vi "polymorphic_addation.vi"   [LabVIEW 2020]
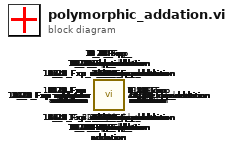
[diagram p0: block diagram]
diagram:
  n1 = call "16_32_Fxp_addation.vi"() -> ()  [unwired: 2 in, 1 out]
  n2 = call "15_32_Fxp_addation.vi"() -> ()  [unwired: 2 in, 1 out]
  n3 = call "14_32_Fxp_addation.vi"() -> ()  [unwired: 2 in, 1 out]
  n4 = call "13_32_Fxp_addation.vi"() -> ()  [unwired: 2 in, 1 out]
  n5 = call "12_32_Fxp_addation.vi"() -> ()  [unwired: 2 in, 1 out]
  n6 = call "11_32_Fxp_addation.vi"() -> ()  [unwired: 2 in, 1 out]
  n7 = call "10_32_Fxp_addation.vi"() -> ()  [unwired: 2 in, 1 out]
  n8 = call "9_32_Fxp_addation.vi"() -> ()  [unwired: 2 in, 1 out]
  n9 = call "8_32_Fxp_addation.vi"() -> ()  [unwired: 2 in, 1 out]
  n10 = call "7_32_Fxp_addation.vi"() -> ()  [unwired: 2 in, 1 out]
  n11 = call "6_32_Fxp_addation.vi"() -> ()  [unwired: 2 in, 1 out]
  n12 = call "5_32_Fxp_addation.vi"() -> ()  [unwired: 2 in, 1 out]
  n13 = call "4_32_Fxp_addation.vi"() -> ()  [unwired: 2 in, 1 out]
  n14 = call "3_32_Fxp_addation.vi"() -> ()  [unwired: 2 in, 1 out]
  n15 = call "2_32_Fxp_addation.vi"() -> ()  [unwired: 2 in, 1 out]
  n16 = call "1_32_Fxp_addation.vi"() -> ()  [unwired: 2 in, 1 out]
  n17 = call "16_31_Fxp_addation.vi"() -> ()  [unwired: 2 in, 1 out]
  n18 = call "15_31_Fxp_addation.vi"() -> ()  [unwired: 2 in, 1 out]
  n19 = call "14_31_Fxp_addation.vi"() -> ()  [unwired: 2 in, 1 out]
  n20 = call "13_31_Fxp_addation.vi"() -> ()  [unwired: 2 in, 1 out]
  n21 = call "12_31_Fxp_addation.vi"() -> ()  [unwired: 2 in, 1 out]
  n22 = call "11_31_Fxp_addation.vi"() -> ()  [unwired: 2 in, 1 out]
  n23 = call "10_31_Fxp_addation.vi"() -> ()  [unwired: 2 in, 1 out]
  n24 = call "9_31_Fxp_addation.vi"() -> ()  [unwired: 2 in, 1 out]
  n25 = call "8_31_Fxp_addation.vi"() -> ()  [unwired: 2 in, 1 out]
  n26 = call "7_31_Fxp_addation.vi"() -> ()  [unwired: 2 in, 1 out]
  n27 = call "6_31_Fxp_addation.vi"() -> ()  [unwired: 2 in, 1 out]
  n28 = call "5_31_Fxp_addation.vi"() -> ()  [unwired: 2 in, 1 out]
  n29 = call "4_31_Fxp_addation.vi"() -> ()  [unwired: 2 in, 1 out]
  n30 = call "3_31_Fxp_addation.vi"() -> ()  [unwired: 2 in, 1 out]
  n31 = call "2_31_Fxp_addation.vi"() -> ()  [unwired: 2 in, 1 out]
  n32 = call "1_31_Fxp_addation.vi"() -> ()  [unwired: 2 in, 1 out]
  n33 = call "16_30_Fxp_addation.vi"() -> ()  [unwired: 2 in, 1 out]
  n34 = call "15_30_Fxp_addation.vi"() -> ()  [unwired: 2 in, 1 out]
  n35 = call "14_30_Fxp_addation.vi"() -> ()  [unwired: 2 in, 1 out]
  n36 = call "13_30_Fxp_addation.vi"() -> ()  [unwired: 2 in, 1 out]
  n37 = call "12_30_Fxp_addation.vi"() -> ()  [unwired: 2 in, 1 out]
  n38 = call "11_30_Fxp_addation.vi"() -> ()  [unwired: 2 in, 1 out]
  n39 = call "10_30_Fxp_addation.vi"() -> ()  [unwired: 2 in, 1 out]
  n40 = call "9_30_Fxp_addation.vi"() -> ()  [unwired: 2 in, 1 out]
  n41 = call "8_30_Fxp_addation.vi"() -> ()  [unwired: 2 in, 1 out]
  n42 = call "7_30_Fxp_addation.vi"() -> ()  [unwired: 2 in, 1 out]
  n43 = call "6_30_Fxp_addation.vi"() -> ()  [unwired: 2 in, 1 out]
  n44 = call "5_30_Fxp_addation.vi"() -> ()  [unwired: 2 in, 1 out]
  n45 = call "4_30_Fxp_addation.vi"() -> ()  [unwired: 2 in, 1 out]
  n46 = call "3_30_Fxp_addation.vi"() -> ()  [unwired: 2 in, 1 out]
  n47 = call "2_30_Fxp_addation.vi"() -> ()  [unwired: 2 in, 1 out]
  n48 = call "1_30_Fxp_addation.vi"() -> ()  [unwired: 2 in, 1 out]
  n49 = call "16_29_Fxp_addation.vi"() -> ()  [unwired: 2 in, 1 out]
  n50 = call "15_29_Fxp_addation.vi"() -> ()  [unwired: 2 in, 1 out]
  n51 = call "14_29_Fxp_addation.vi"() -> ()  [unwired: 2 in, 1 out]
  n52 = call "13_29_Fxp_addation.vi"() -> ()  [unwired: 2 in, 1 out]
  n53 = call "12_29_Fxp_addation.vi"() -> ()  [unwired: 2 in, 1 out]
  n54 = call "11_29_Fxp_addation.vi"() -> ()  [unwired: 2 in, 1 out]
  n55 = call "10_29_Fxp_addation.vi"() -> ()  [unwired: 2 in, 1 out]
  n56 = call "9_29_Fxp_addation.vi"() -> ()  [unwired: 2 in, 1 out]
  n57 = call "8_29_Fxp_addation.vi"() -> ()  [unwired: 2 in, 1 out]
  n58 = call "7_29_Fxp_addation.vi"() -> ()  [unwired: 2 in, 1 out]
  n59 = call "6_29_Fxp_addation.vi"() -> ()  [unwired: 2 in, 1 out]
  n60 = call "5_29_Fxp_addation.vi"() -> ()  [unwired: 2 in, 1 out]
  n61 = call "4_29_Fxp_addation.vi"() -> ()  [unwired: 2 in, 1 out]
  n62 = call "3_29_Fxp_addation.vi"() -> ()  [unwired: 2 in, 1 out]
  n63 = call "2_29_Fxp_addation.vi"() -> ()  [unwired: 2 in, 1 out]
  n64 = call "1_29_Fxp_addation.vi"() -> ()  [unwired: 2 in, 1 out]
  n65 = call "16_28_Fxp_addation.vi"() -> ()  [unwired: 2 in, 1 out]
  n66 = call "15_28_Fxp_addation.vi"() -> ()  [unwired: 2 in, 1 out]
  n67 = call "14_28_Fxp_addation.vi"() -> ()  [unwired: 2 in, 1 out]
  n68 = call "13_28_Fxp_addation.vi"() -> ()  [unwired: 2 in, 1 out]
  n69 = call "12_28_Fxp_addation.vi"() -> ()  [unwired: 2 in, 1 out]
  n70 = call "11_28_Fxp_addation.vi"() -> ()  [unwired: 2 in, 1 out]
  n71 = call "10_28_Fxp_addation.vi"() -> ()  [unwired: 2 in, 1 out]
  n72 = call "9_28_Fxp_addation.vi"() -> ()  [unwired: 2 in, 1 out]
  n73 = call "8_28_Fxp_addation.vi"() -> ()  [unwired: 2 in, 1 out]
  n74 = call "7_28_Fxp_addation.vi"() -> ()  [unwired: 2 in, 1 out]
  n75 = call "6_28_Fxp_addation.vi"() -> ()  [unwired: 2 in, 1 out]
  n76 = call "5_28_Fxp_addation.vi"() -> ()  [unwired: 2 in, 1 out]
  n77 = call "4_28_Fxp_addation.vi"() -> ()  [unwired: 2 in, 1 out]
  n78 = call "3_28_Fxp_addation.vi"() -> ()  [unwired: 2 in, 1 out]
  n79 = call "2_28_Fxp_addation.vi"() -> ()  [unwired: 2 in, 1 out]
  n80 = call "1_28_Fxp_addation.vi"() -> ()  [unwired: 2 in, 1 out]
  n81 = call "16_27_Fxp_addation.vi"() -> ()  [unwired: 2 in, 1 out]
  n82 = call "15_27_Fxp_addation.vi"() -> ()  [unwired: 2 in, 1 out]
  n83 = call "14_27_Fxp_addation.vi"() -> ()  [unwired: 2 in, 1 out]
  n84 = call "13_27_Fxp_addation.vi"() -> ()  [unwired: 2 in, 1 out]
  n85 = call "12_27_Fxp_addation.vi"() -> ()  [unwired: 2 in, 1 out]
  n86 = call "11_27_Fxp_addation.vi"() -> ()  [unwired: 2 in, 1 out]
  n87 = call "10_27_Fxp_addation.vi"() -> ()  [unwired: 2 in, 1 out]
  n88 = call "9_27_Fxp_addation.vi"() -> ()  [unwired: 2 in, 1 out]
  n89 = call "8_27_Fxp_addation.vi"() -> ()  [unwired: 2 in, 1 out]
  n90 = call "7_27_Fxp_addation.vi"() -> ()  [unwired: 2 in, 1 out]
  n91 = call "6_27_Fxp_addation.vi"() -> ()  [unwired: 2 in, 1 out]
  n92 = call "5_27_Fxp_addation.vi"() -> ()  [unwired: 2 in, 1 out]
  n93 = call "4_27_Fxp_addation.vi"() -> ()  [unwired: 2 in, 1 out]
  n94 = call "3_27_Fxp_addation.vi"() -> ()  [unwired: 2 in, 1 out]
  n95 = call "2_27_Fxp_addation.vi"() -> ()  [unwired: 2 in, 1 out]
  n96 = call "1_27_Fxp_addation.vi"() -> ()  [unwired: 2 in, 1 out]
  n97 = call "16_26_Fxp_addation.vi"() -> ()  [unwired: 2 in, 1 out]
  n98 = call "15_26_Fxp_addation.vi"() -> ()  [unwired: 2 in, 1 out]
  n99 = call "14_26_Fxp_addation.vi"() -> ()  [unwired: 2 in, 1 out]
  n100 = call "13_26_Fxp_addation.vi"() -> ()  [unwired: 2 in, 1 out]
  n101 = call "12_26_Fxp_addation.vi"() -> ()  [unwired: 2 in, 1 out]
  n102 = call "11_26_Fxp_addation.vi"() -> ()  [unwired: 2 in, 1 out]
  n103 = call "10_26_Fxp_addation.vi"() -> ()  [unwired: 2 in, 1 out]
  n104 = call "9_26_Fxp_addation.vi"() -> ()  [unwired: 2 in, 1 out]
  n105 = call "8_26_Fxp_addation.vi"() -> ()  [unwired: 2 in, 1 out]
  n106 = call "7_26_Fxp_addation.vi"() -> ()  [unwired: 2 in, 1 out]
  n107 = call "6_26_Fxp_addation.vi"() -> ()  [unwired: 2 in, 1 out]
  n108 = call "5_26_Fxp_addation.vi"() -> ()  [unwired: 2 in, 1 out]
  n109 = call "4_26_Fxp_addation.vi"() -> ()  [unwired: 2 in, 1 out]
  n110 = call "3_26_Fxp_addation.vi"() -> ()  [unwired: 2 in, 1 out]
  n111 = call "2_26_Fxp_addation.vi"() -> ()  [unwired: 2 in, 1 out]
  n112 = call "1_26_Fxp_addation.vi"() -> ()  [unwired: 2 in, 1 out]
  n113 = call "16_25_Fxp_addation.vi"() -> ()  [unwired: 2 in, 1 out]
  n114 = call "15_25_Fxp_addation.vi"() -> ()  [unwired: 2 in, 1 out]
  n115 = call "14_25_Fxp_addation.vi"() -> ()  [unwired: 2 in, 1 out]
  n116 = call "13_25_Fxp_addation.vi"() -> ()  [unwired: 2 in, 1 out]
  n117 = call "12_25_Fxp_addation.vi"() -> ()  [unwired: 2 in, 1 out]
  n118 = call "11_25_Fxp_addation.vi"() -> ()  [unwired: 2 in, 1 out]
  n119 = call "10_25_Fxp_addation.vi"() -> ()  [unwired: 2 in, 1 out]
  n120 = call "9_25_Fxp_addation.vi"() -> ()  [unwired: 2 in, 1 out]
  n121 = call "8_25_Fxp_addation.vi"() -> ()  [unwired: 2 in, 1 out]
  n122 = call "7_25_Fxp_addation.vi"() -> ()  [unwired: 2 in, 1 out]
  n123 = call "6_25_Fxp_addation.vi"() -> ()  [unwired: 2 in, 1 out]
  n124 = call "5_25_Fxp_addation.vi"() -> ()  [unwired: 2 in, 1 out]
  n125 = call "4_25_Fxp_addation.vi"() -> ()  [unwired: 2 in, 1 out]
  n126 = call "3_25_Fxp_addation.vi"() -> ()  [unwired: 2 in, 1 out]
  n127 = call "2_25_Fxp_addation.vi"() -> ()  [unwired: 2 in, 1 out]
  n128 = call "1_25_Fxp_addation.vi"() -> ()  [unwired: 2 in, 1 out]
  n129 = call "16_24_Fxp_addation.vi"() -> ()  [unwired: 2 in, 1 out]
  n130 = call "15_24_Fxp_addation.vi"() -> ()  [unwired: 2 in, 1 out]
  n131 = call "14_24_Fxp_addation.vi"() -> ()  [unwired: 2 in, 1 out]
  n132 = call "13_24_Fxp_addation.vi"() -> ()  [unwired: 2 in, 1 out]
  n133 = call "12_24_Fxp_addation.vi"() -> ()  [unwired: 2 in, 1 out]
  n134 = call "11_24_Fxp_addation.vi"() -> ()  [unwired: 2 in, 1 out]
  n135 = call "10_24_Fxp_addation.vi"() -> ()  [unwired: 2 in, 1 out]
  n136 = call "9_24_Fxp_addation.vi"() -> ()  [unwired: 2 in, 1 out]
  n137 = call "8_24_Fxp_addation.vi"() -> ()  [unwired: 2 in, 1 out]
  n138 = call "7_24_Fxp_addation.vi"() -> ()  [unwired: 2 in, 1 out]
  n139 = call "6_24_Fxp_addation.vi"() -> ()  [unwired: 2 in, 1 out]
  n140 = call "5_24_Fxp_addation.vi"() -> ()  [unwired: 2 in, 1 out]
  n141 = call "4_24_Fxp_addation.vi"() -> ()  [unwired: 2 in, 1 out]
  n142 = call "3_24_Fxp_addation.vi"() -> ()  [unwired: 2 in, 1 out]
  n143 = call "2_24_Fxp_addation.vi"() -> ()  [unwired: 2 in, 1 out]
  n144 = call "1_24_Fxp_addation.vi"() -> ()  [unwired: 2 in, 1 out]
  n145 = call "16_23_Fxp_addation.vi"() -> ()  [unwired: 2 in, 1 out]
  n146 = call "15_23_Fxp_addation.vi"() -> ()  [unwired: 2 in, 1 out]
  n147 = call "14_23_Fxp_addation.vi"() -> ()  [unwired: 2 in, 1 out]
  n148 = call "13_23_Fxp_addation.vi"() -> ()  [unwired: 2 in, 1 out]
  n149 = call "12_23_Fxp_addation.vi"() -> ()  [unwired: 2 in, 1 out]
  n150 = call "11_23_Fxp_addation.vi"() -> ()  [unwired: 2 in, 1 out]
  n151 = call "10_23_Fxp_addation.vi"() -> ()  [unwired: 2 in, 1 out]
  n152 = call "9_23_Fxp_addation.vi"() -> ()  [unwired: 2 in, 1 out]
  n153 = call "8_23_Fxp_addation.vi"() -> ()  [unwired: 2 in, 1 out]
  n154 = call "7_23_Fxp_addation.vi"() -> ()  [unwired: 2 in, 1 out]
  n155 = call "6_23_Fxp_addation.vi"() -> ()  [unwired: 2 in, 1 out]
  n156 = call "5_23_Fxp_addation.vi"() -> ()  [unwired: 2 in, 1 out]
  n157 = call "4_23_Fxp_addation.vi"() -> ()  [unwired: 2 in, 1 out]
  n158 = call "3_23_Fxp_addation.vi"() -> ()  [unwired: 2 in, 1 out]
  n159 = call "2_23_Fxp_addation.vi"() -> ()  [unwired: 2 in, 1 out]
  n160 = call "1_23_Fxp_addation.vi"() -> ()  [unwired: 2 in, 1 out]
  n161 = call "16_22_Fxp_addation.vi"() -> ()  [unwired: 2 in, 1 out]
  n162 = call "15_22_Fxp_addation.vi"() -> ()  [unwired: 2 in, 1 out]
  n163 = call "14_22_Fxp_addation.vi"() -> ()  [unwired: 2 in, 1 out]
  n164 = call "13_22_Fxp_addation.vi"() -> ()  [unwired: 2 in, 1 out]
  n165 = call "12_22_Fxp_addation.vi"() -> ()  [unwired: 2 in, 1 out]
  n166 = call "11_22_Fxp_addation.vi"() -> ()  [unwired: 2 in, 1 out]
  n167 = call "10_22_Fxp_addation.vi"() -> ()  [unwired: 2 in, 1 out]
  n168 = call "9_22_Fxp_addation.vi"() -> ()  [unwired: 2 in, 1 out]
  n169 = call "8_22_Fxp_addation.vi"() -> ()  [unwired: 2 in, 1 out]
  n170 = call "7_22_Fxp_addation.vi"() -> ()  [unwired: 2 in, 1 out]
  n171 = call "6_22_Fxp_addation.vi"() -> ()  [unwired: 2 in, 1 out]
  n172 = call "5_22_Fxp_addation.vi"() -> ()  [unwired: 2 in, 1 out]
  n173 = call "4_22_Fxp_addation.vi"() -> ()  [unwired: 2 in, 1 out]
  n174 = call "3_22_Fxp_addation.vi"() -> ()  [unwired: 2 in, 1 out]
  n175 = call "2_22_Fxp_addation.vi"() -> ()  [unwired: 2 in, 1 out]
  n176 = call "1_22_Fxp_addation.vi"() -> ()  [unwired: 2 in, 1 out]
  n177 = call "16_21_Fxp_addation.vi"() -> ()  [unwired: 2 in, 1 out]
  n178 = call "15_21_Fxp_addation.vi"() -> ()  [unwired: 2 in, 1 out]
  n179 = call "14_21_Fxp_addation.vi"() -> ()  [unwired: 2 in, 1 out]
  n180 = call "13_21_Fxp_addation.vi"() -> ()  [unwired: 2 in, 1 out]
  n181 = call "12_21_Fxp_addation.vi"() -> ()  [unwired: 2 in, 1 out]
  n182 = call "11_21_Fxp_addation.vi"() -> ()  [unwired: 2 in, 1 out]
  n183 = call "10_21_Fxp_addation.vi"() -> ()  [unwired: 2 in, 1 out]
  n184 = call "9_21_Fxp_addation.vi"() -> ()  [unwired: 2 in, 1 out]
  n185 = call "8_21_Fxp_addation.vi"() -> ()  [unwired: 2 in, 1 out]
  n186 = call "7_21_Fxp_addation.vi"() -> ()  [unwired: 2 in, 1 out]
  n187 = call "6_21_Fxp_addation.vi"() -> ()  [unwired: 2 in, 1 out]
  n188 = call "5_21_Fxp_addation.vi"() -> ()  [unwired: 2 in, 1 out]
  n189 = call "4_21_Fxp_addation.vi"() -> ()  [unwired: 2 in, 1 out]
  n190 = call "3_21_Fxp_addation.vi"() -> ()  [unwired: 2 in, 1 out]
  n191 = call "2_21_Fxp_addation.vi"() -> ()  [unwired: 2 in, 1 out]
  n192 = call "1_21_Fxp_addation.vi"() -> ()  [unwired: 2 in, 1 out]
  n193 = call "16_20_Fxp_addation.vi"() -> ()  [unwired: 2 in, 1 out]
  n194 = call "15_20_Fxp_addation.vi"() -> ()  [unwired: 2 in, 1 out]
  n195 = call "14_20_Fxp_addation.vi"() -> ()  [unwired: 2 in, 1 out]
  n196 = call "13_20_Fxp_addation.vi"() -> ()  [unwired: 2 in, 1 out]
  n197 = call "12_20_Fxp_addation.vi"() -> ()  [unwired: 2 in, 1 out]
  n198 = call "11_20_Fxp_addation.vi"() -> ()  [unwired: 2 in, 1 out]
  n199 = call "10_20_Fxp_addation.vi"() -> ()  [unwired: 2 in, 1 out]
  n200 = call "9_20_Fxp_addation.vi"() -> ()  [unwired: 2 in, 1 out]
  n201 = call "8_20_Fxp_addation.vi"() -> ()  [unwired: 2 in, 1 out]
  n202 = call "7_20_Fxp_addation.vi"() -> ()  [unwired: 2 in, 1 out]
  n203 = call "6_20_Fxp_addation.vi"() -> ()  [unwired: 2 in, 1 out]
  n204 = call "5_20_Fxp_addation.vi"() -> ()  [unwired: 2 in, 1 out]
  n205 = call "4_20_Fxp_addation.vi"() -> ()  [unwired: 2 in, 1 out]
  n206 = call "3_20_Fxp_addation.vi"() -> ()  [unwired: 2 in, 1 out]
  n207 = call "2_20_Fxp_addation.vi"() -> ()  [unwired: 2 in, 1 out]
  n208 = call "1_20_Fxp_addation.vi"() -> ()  [unwired: 2 in, 1 out]
  n209 = call "16_19_Fxp_addation.vi"() -> ()  [unwired: 2 in, 1 out]
  n210 = call "15_19_Fxp_addation.vi"() -> ()  [unwired: 2 in, 1 out]
  n211 = call "14_19_Fxp_addation.vi"() -> ()  [unwired: 2 in, 1 out]
  n212 = call "13_19_Fxp_addation.vi"() -> ()  [unwired: 2 in, 1 out]
  n213 = call "12_19_Fxp_addation.vi"() -> ()  [unwired: 2 in, 1 out]
  n214 = call "11_19_Fxp_addation.vi"() -> ()  [unwired: 2 in, 1 out]
  n215 = call "10_19_Fxp_addation.vi"() -> ()  [unwired: 2 in, 1 out]
  n216 = call "9_19_Fxp_addation.vi"() -> ()  [unwired: 2 in, 1 out]
  n217 = call "8_19_Fxp_addation.vi"() -> ()  [unwired: 2 in, 1 out]
  n218 = call "7_19_Fxp_addation.vi"() -> ()  [unwired: 2 in, 1 out]
  n219 = call "6_19_Fxp_addation.vi"() -> ()  [unwired: 2 in, 1 out]
  n220 = call "5_19_Fxp_addation.vi"() -> ()  [unwired: 2 in, 1 out]
  n221 = call "4_19_Fxp_addation.vi"() -> ()  [unwired: 2 in, 1 out]
  n222 = call "3_19_Fxp_addation.vi"() -> ()  [unwired: 2 in, 1 out]
  n223 = call "2_19_Fxp_addation.vi"() -> ()  [unwired: 2 in, 1 out]
  n224 = call "1_19_Fxp_addation.vi"() -> ()  [unwired: 2 in, 1 out]
  n225 = call "16_18_Fxp_addation.vi"() -> ()  [unwired: 2 in, 1 out]
  n226 = call "15_18_Fxp_addation.vi"() -> ()  [unwired: 2 in, 1 out]
  n227 = call "14_18_Fxp_addation.vi"() -> ()  [unwired: 2 in, 1 out]
  n228 = call "13_18_Fxp_addation.vi"() -> ()  [unwired: 2 in, 1 out]
  n229 = call "12_18_Fxp_addation.vi"() -> ()  [unwired: 2 in, 1 out]
  n230 = call "11_18_Fxp_addation.vi"() -> ()  [unwired: 2 in, 1 out]
  n231 = call "10_18_Fxp_addation.vi"() -> ()  [unwired: 2 in, 1 out]
  n232 = call "9_18_Fxp_addation.vi"() -> ()  [unwired: 2 in, 1 out]
  n233 = call "8_18_Fxp_addation.vi"() -> ()  [unwired: 2 in, 1 out]
  n234 = call "7_18_Fxp_addation.vi"() -> ()  [unwired: 2 in, 1 out]
  n235 = call "6_18_Fxp_addation.vi"() -> ()  [unwired: 2 in, 1 out]
  n236 = call "5_18_Fxp_addation.vi"() -> ()  [unwired: 2 in, 1 out]
  n237 = call "4_18_Fxp_addation.vi"() -> ()  [unwired: 2 in, 1 out]
  n238 = call "3_18_Fxp_addation.vi"() -> ()  [unwired: 2 in, 1 out]
  n239 = call "2_18_Fxp_addation.vi"() -> ()  [unwired: 2 in, 1 out]
  n240 = call "1_18_Fxp_addation.vi"() -> ()  [unwired: 2 in, 1 out]
  n241 = call "16_17_Fxp_addation.vi"() -> ()  [unwired: 2 in, 1 out]
  n242 = call "15_17_Fxp_addation.vi"() -> ()  [unwired: 2 in, 1 out]
  n243 = call "14_17_Fxp_addation.vi"() -> ()  [unwired: 2 in, 1 out]
  n244 = call "13_17_Fxp_addation.vi"() -> ()  [unwired: 2 in, 1 out]
  n245 = call "12_17_Fxp_addation.vi"() -> ()  [unwired: 2 in, 1 out]
  n246 = call "11_17_Fxp_addation.vi"() -> ()  [unwired: 2 in, 1 out]
  n247 = call "10_17_Fxp_addation.vi"() -> ()  [unwired: 2 in, 1 out]
  n248 = call "9_17_Fxp_addation.vi"() -> ()  [unwired: 2 in, 1 out]
  n249 = call "8_17_Fxp_addation.vi"() -> ()  [unwired: 2 in, 1 out]
  n250 = call "7_17_Fxp_addation.vi"() -> ()  [unwired: 2 in, 1 out]
  n251 = call "6_17_Fxp_addation.vi"() -> ()  [unwired: 2 in, 1 out]
  n252 = call "5_17_Fxp_addation.vi"() -> ()  [unwired: 2 in, 1 out]
  n253 = call "4_17_Fxp_addation.vi"() -> ()  [unwired: 2 in, 1 out]
  n254 = call "3_17_Fxp_addation.vi"() -> ()  [unwired: 2 in, 1 out]
  n255 = call "2_17_Fxp_addation.vi"() -> ()  [unwired: 2 in, 1 out]
  n256 = call "1_17_Fxp_addation.vi"() -> ()  [unwired: 2 in, 1 out]
  n257 = call "16_16_Fxp_addation.vi"() -> ()  [unwired: 2 in, 1 out]
  n258 = call "15_16_Fxp_addation.vi"() -> ()  [unwired: 2 in, 1 out]
  n259 = call "14_16_Fxp_addation.vi"() -> ()  [unwired: 2 in, 1 out]
  n260 = call "13_16_Fxp_addation.vi"() -> ()  [unwired: 2 in, 1 out]
  n261 = call "12_16_Fxp_addation.vi"() -> ()  [unwired: 2 in, 1 out]
  n262 = call "11_16_Fxp_addation.vi"() -> ()  [unwired: 2 in, 1 out]
  n263 = call "10_16_Fxp_addation.vi"() -> ()  [unwired: 2 in, 1 out]
  n264 = call "9_16_Fxp_addation.vi"() -> ()  [unwired: 2 in, 1 out]
  n265 = call "8_16_Fxp_addation.vi"() -> ()  [unwired: 2 in, 1 out]
  n266 = call "7_16_Fxp_addation.vi"() -> ()  [unwired: 2 in, 1 out]
  n267 = call "6_16_Fxp_addation.vi"() -> ()  [unwired: 2 in, 1 out]
  n268 = call "5_16_Fxp_addation.vi"() -> ()  [unwired: 2 in, 1 out]
  n269 = call "4_16_Fxp_addation.vi"() -> ()  [unwired: 2 in, 1 out]
  n270 = call "3_16_Fxp_addation.vi"() -> ()  [unwired: 2 in, 1 out]
  n271 = call "2_16_Fxp_addation.vi"() -> ()  [unwired: 2 in, 1 out]
  n272 = call "1_16_Fxp_addation.vi"() -> ()  [unwired: 2 in, 1 out]
  n273 = call "16_15_Fxp_addation.vi"() -> ()  [unwired: 2 in, 1 out]
  n274 = call "15_15_Fxp_addation.vi"() -> ()  [unwired: 2 in, 1 out]
  n275 = call "14_15_Fxp_addation.vi"() -> ()  [unwired: 2 in, 1 out]
  n276 = call "13_15_Fxp_addation.vi"() -> ()  [unwired: 2 in, 1 out]
  n277 = call "12_15_Fxp_addation.vi"() -> ()  [unwired: 2 in, 1 out]
  n278 = call "11_15_Fxp_addation.vi"() -> ()  [unwired: 2 in, 1 out]
  n279 = call "10_15_Fxp_addation.vi"() -> ()  [unwired: 2 in, 1 out]
  n280 = call "9_15_Fxp_addation.vi"() -> ()  [unwired: 2 in, 1 out]
  n281 = call "8_15_Fxp_addation.vi"() -> ()  [unwired: 2 in, 1 out]
  n282 = call "7_15_Fxp_addation.vi"() -> ()  [unwired: 2 in, 1 out]
  n283 = call "6_15_Fxp_addation.vi"() -> ()  [unwired: 2 in, 1 out]
  n284 = call "5_15_Fxp_addation.vi"() -> ()  [unwired: 2 in, 1 out]
  n285 = call "4_15_Fxp_addation.vi"() -> ()  [unwired: 2 in, 1 out]
  n286 = call "3_15_Fxp_addation.vi"() -> ()  [unwired: 2 in, 1 out]
  n287 = call "2_15_Fxp_addation.vi"() -> ()  [unwired: 2 in, 1 out]
  n288 = call "1_15_Fxp_addation.vi"() -> ()  [unwired: 2 in, 1 out]
  n289 = call "16_14_Fxp_addation.vi"() -> ()  [unwired: 2 in, 1 out]
  n290 = call "15_14_Fxp_addation.vi"() -> ()  [unwired: 2 in, 1 out]
  n291 = call "14_14_Fxp_addation.vi"() -> ()  [unwired: 2 in, 1 out]
  n292 = call "13_14_Fxp_addation.vi"() -> ()  [unwired: 2 in, 1 out]
  n293 = call "12_14_Fxp_addation.vi"() -> ()  [unwired: 2 in, 1 out]
  n294 = call "11_14_Fxp_addation.vi"() -> ()  [unwired: 2 in, 1 out]
  n295 = call "10_14_Fxp_addation.vi"() -> ()  [unwired: 2 in, 1 out]
  n296 = call "9_14_Fxp_addation.vi"() -> ()  [unwired: 2 in, 1 out]
  n297 = call "8_14_Fxp_addation.vi"() -> ()  [unwired: 2 in, 1 out]
  n298 = call "7_14_Fxp_addation.vi"() -> ()  [unwired: 2 in, 1 out]
  n299 = call "6_14_Fxp_addation.vi"() -> ()  [unwired: 2 in, 1 out]
  n300 = call "5_14_Fxp_addation.vi"() -> ()  [unwired: 2 in, 1 out]
  n301 = call "4_14_Fxp_addation.vi"() -> ()  [unwired: 2 in, 1 out]
  n302 = call "3_14_Fxp_addation.vi"() -> ()  [unwired: 2 in, 1 out]
  n303 = call "2_14_Fxp_addation.vi"() -> ()  [unwired: 2 in, 1 out]
  n304 = call "1_14_Fxp_addation.vi"() -> ()  [unwired: 2 in, 1 out]
  n305 = call "16_13_Fxp_addation.vi"() -> ()  [unwired: 2 in, 1 out]
  n306 = call "15_13_Fxp_addation.vi"() -> ()  [unwired: 2 in, 1 out]
  n307 = call "14_13_Fxp_addation.vi"() -> ()  [unwired: 2 in, 1 out]
  n308 = call "13_13_Fxp_addation.vi"() -> ()  [unwired: 2 in, 1 out]
  n309 = call "12_13_Fxp_addation.vi"() -> ()  [unwired: 2 in, 1 out]
  n310 = call "11_13_Fxp_addation.vi"() -> ()  [unwired: 2 in, 1 out]
  n311 = call "10_13_Fxp_addation.vi"() -> ()  [unwired: 2 in, 1 out]
  n312 = call "9_13_Fxp_addation.vi"() -> ()  [unwired: 2 in, 1 out]
  n313 = call "8_13_Fxp_addation.vi"() -> ()  [unwired: 2 in, 1 out]
  n314 = call "7_13_Fxp_addation.vi"() -> ()  [unwired: 2 in, 1 out]
  n315 = call "6_13_Fxp_addation.vi"() -> ()  [unwired: 2 in, 1 out]
  n316 = call "5_13_Fxp_addation.vi"() -> ()  [unwired: 2 in, 1 out]
  n317 = call "4_13_Fxp_addation.vi"() -> ()  [unwired: 2 in, 1 out]
  n318 = call "3_13_Fxp_addation.vi"() -> ()  [unwired: 2 in, 1 out]
  n319 = call "2_13_Fxp_addation.vi"() -> ()  [unwired: 2 in, 1 out]
  n320 = call "1_13_Fxp_addation.vi"() -> ()  [unwired: 2 in, 1 out]
  n321 = call "16_12_Fxp_addation.vi"() -> ()  [unwired: 2 in, 1 out]
  n322 = call "15_12_Fxp_addation.vi"() -> ()  [unwired: 2 in, 1 out]
  n323 = call "14_12_Fxp_addation.vi"() -> ()  [unwired: 2 in, 1 out]
  n324 = call "13_12_Fxp_addation.vi"() -> ()  [unwired: 2 in, 1 out]
  n325 = call "12_12_Fxp_addation.vi"() -> ()  [unwired: 2 in, 1 out]
  n326 = call "11_12_Fxp_addation.vi"() -> ()  [unwired: 2 in, 1 out]
  n327 = call "10_12_Fxp_addation.vi"() -> ()  [unwired: 2 in, 1 out]
  n328 = call "9_12_Fxp_addation.vi"() -> ()  [unwired: 2 in, 1 out]
  n329 = call "8_12_Fxp_addation.vi"() -> ()  [unwired: 2 in, 1 out]
  n330 = call "7_12_Fxp_addation.vi"() -> ()  [unwired: 2 in, 1 out]
  n331 = call "6_12_Fxp_addation.vi"() -> ()  [unwired: 2 in, 1 out]
  n332 = call "5_12_Fxp_addation.vi"() -> ()  [unwired: 2 in, 1 out]
  n333 = call "4_12_Fxp_addation.vi"() -> ()  [unwired: 2 in, 1 out]
  n334 = call "3_12_Fxp_addation.vi"() -> ()  [unwired: 2 in, 1 out]
  n335 = call "2_12_Fxp_addation.vi"() -> ()  [unwired: 2 in, 1 out]
  n336 = call "1_12_Fxp_addation.vi"() -> ()  [unwired: 2 in, 1 out]
  n337 = call "16_11_Fxp_addation.vi"() -> ()  [unwired: 2 in, 1 out]
  n338 = call "15_11_Fxp_addation.vi"() -> ()  [unwired: 2 in, 1 out]
  n339 = call "14_11_Fxp_addation.vi"() -> ()  [unwired: 2 in, 1 out]
  n340 = call "13_11_Fxp_addation.vi"() -> ()  [unwired: 2 in, 1 out]
  n341 = call "12_11_Fxp_addation.vi"() -> ()  [unwired: 2 in, 1 out]
  n342 = call "11_11_Fxp_addation.vi"() -> ()  [unwired: 2 in, 1 out]
  n343 = call "10_11_Fxp_addation.vi"() -> ()  [unwired: 2 in, 1 out]
  n344 = call "9_11_Fxp_addation.vi"() -> ()  [unwired: 2 in, 1 out]
  n345 = call "8_11_Fxp_addation.vi"() -> ()  [unwired: 2 in, 1 out]
  n346 = call "7_11_Fxp_addation.vi"() -> ()  [unwired: 2 in, 1 out]
  n347 = call "6_11_Fxp_addation.vi"() -> ()  [unwired: 2 in, 1 out]
  n348 = call "5_11_Fxp_addation.vi"() -> ()  [unwired: 2 in, 1 out]
  n349 = call "4_11_Fxp_addation.vi"() -> ()  [unwired: 2 in, 1 out]
  n350 = call "3_11_Fxp_addation.vi"() -> ()  [unwired: 2 in, 1 out]
  n351 = call "2_11_Fxp_addation.vi"() -> ()  [unwired: 2 in, 1 out]
  n352 = call "1_11_Fxp_addation.vi"() -> ()  [unwired: 2 in, 1 out]
  n353 = call "16_10_Fxp_addation.vi"() -> ()  [unwired: 2 in, 1 out]
  n354 = call "15_10_Fxp_addation.vi"() -> ()  [unwired: 2 in, 1 out]
  n355 = call "14_10_Fxp_addation.vi"() -> ()  [unwired: 2 in, 1 out]
  n356 = call "13_10_Fxp_addation.vi"() -> ()  [unwired: 2 in, 1 out]
  n357 = call "12_10_Fxp_addation.vi"() -> ()  [unwired: 2 in, 1 out]
  n358 = call "11_10_Fxp_addation.vi"() -> ()  [unwired: 2 in, 1 out]
  n359 = call "10_10_Fxp_addation.vi"() -> ()  [unwired: 2 in, 1 out]
  n360 = call "9_10_Fxp_addation.vi"() -> ()  [unwired: 2 in, 1 out]
  n361 = call "8_10_Fxp_addation.vi"() -> ()  [unwired: 2 in, 1 out]
  n362 = call "7_10_Fxp_addation.vi"() -> ()  [unwired: 2 in, 1 out]
  n363 = call "6_10_Fxp_addation.vi"() -> ()  [unwired: 2 in, 1 out]
  n364 = call "5_10_Fxp_addation.vi"() -> ()  [unwired: 2 in, 1 out]
  n365 = call "4_10_Fxp_addation.vi"() -> ()  [unwired: 2 in, 1 out]
  n366 = call "3_10_Fxp_addation.vi"() -> ()  [unwired: 2 in, 1 out]
  n367 = call "2_10_Fxp_addation.vi"() -> ()  [unwired: 2 in, 1 out]
  n368 = call "1_10_Fxp_addation.vi"() -> ()  [unwired: 2 in, 1 out]
  n369 = call "16_9_Fxp_addation.vi"() -> ()  [unwired: 2 in, 1 out]
  n370 = call "15_9_Fxp_addation.vi"() -> ()  [unwired: 2 in, 1 out]
  n371 = call "14_9_Fxp_addation.vi"() -> ()  [unwired: 2 in, 1 out]
  n372 = call "13_9_Fxp_addation.vi"() -> ()  [unwired: 2 in, 1 out]
  n373 = call "12_9_Fxp_addation.vi"() -> ()  [unwired: 2 in, 1 out]
  n374 = call "11_9_Fxp_addation.vi"() -> ()  [unwired: 2 in, 1 out]
  n375 = call "10_9_Fxp_addation.vi"() -> ()  [unwired: 2 in, 1 out]
  n376 = call "9_9_Fxp_addation.vi"() -> ()  [unwired: 2 in, 1 out]
  n377 = call "8_9_Fxp_addation.vi"() -> ()  [unwired: 2 in, 1 out]
  n378 = call "7_9_Fxp_addation.vi"() -> ()  [unwired: 2 in, 1 out]
  n379 = call "6_9_Fxp_addation.vi"() -> ()  [unwired: 2 in, 1 out]
  n380 = call "5_9_Fxp_addation.vi"() -> ()  [unwired: 2 in, 1 out]
  n381 = call "4_9_Fxp_addation.vi"() -> ()  [unwired: 2 in, 1 out]
  n382 = call "3_9_Fxp_addation.vi"() -> ()  [unwired: 2 in, 1 out]
  n383 = call "2_9_Fxp_addation.vi"() -> ()  [unwired: 2 in, 1 out]
  n384 = call "1_9_Fxp_addation.vi"() -> ()  [unwired: 2 in, 1 out]
  n385 = call "16_8_Fxp_addation.vi"() -> ()  [unwired: 2 in, 1 out]
  n386 = call "15_8_Fxp_addation.vi"() -> ()  [unwired: 2 in, 1 out]
  n387 = call "14_8_Fxp_addation.vi"() -> ()  [unwired: 2 in, 1 out]
  n388 = call "13_8_Fxp_addation.vi"() -> ()  [unwired: 2 in, 1 out]
  n389 = call "12_8_Fxp_addation.vi"() -> ()  [unwired: 2 in, 1 out]
  n390 = call "11_8_Fxp_addation.vi"() -> ()  [unwired: 2 in, 1 out]
  n391 = call "10_8_Fxp_addation.vi"() -> ()  [unwired: 2 in, 1 out]
  n392 = call "9_8_Fxp_addation.vi"() -> ()  [unwired: 2 in, 1 out]
  n393 = call "8_8_Fxp_addation.vi"() -> ()  [unwired: 2 in, 1 out]
  n394 = call "7_8_Fxp_addation.vi"() -> ()  [unwired: 2 in, 1 out]
  n395 = call "6_8_Fxp_addation.vi"() -> ()  [unwired: 2 in, 1 out]
  n396 = call "5_8_Fxp_addation.vi"() -> ()  [unwired: 2 in, 1 out]
  n397 = call "4_8_Fxp_addation.vi"() -> ()  [unwired: 2 in, 1 out]
  n398 = call "3_8_Fxp_addation.vi"() -> ()  [unwired: 2 in, 1 out]
  n399 = call "2_8_Fxp_addation.vi"() -> ()  [unwired: 2 in, 1 out]
  n400 = call "1_8_Fxp_addation.vi"() -> ()  [unwired: 2 in, 1 out]
  n401 = call "16_7_Fxp_addation.vi"() -> ()  [unwired: 2 in, 1 out]
  n402 = call "15_7_Fxp_addation.vi"() -> ()  [unwired: 2 in, 1 out]
  n403 = call "14_7_Fxp_addation.vi"() -> ()  [unwired: 2 in, 1 out]
  n404 = call "13_7_Fxp_addation.vi"() -> ()  [unwired: 2 in, 1 out]
  n405 = call "12_7_Fxp_addation.vi"() -> ()  [unwired: 2 in, 1 out]
  n406 = call "11_7_Fxp_addation.vi"() -> ()  [unwired: 2 in, 1 out]
  n407 = call "10_7_Fxp_addation.vi"() -> ()  [unwired: 2 in, 1 out]
  n408 = call "9_7_Fxp_addation.vi"() -> ()  [unwired: 2 in, 1 out]
  n409 = call "8_7_Fxp_addation.vi"() -> ()  [unwired: 2 in, 1 out]
  n410 = call "7_7_Fxp_addation.vi"() -> ()  [unwired: 2 in, 1 out]
  n411 = call "6_7_Fxp_addation.vi"() -> ()  [unwired: 2 in, 1 out]
  n412 = call "5_7_Fxp_addation.vi"() -> ()  [unwired: 2 in, 1 out]
  n413 = call "4_7_Fxp_addation.vi"() -> ()  [unwired: 2 in, 1 out]
  n414 = call "3_7_Fxp_addation.vi"() -> ()  [unwired: 2 in, 1 out]
  n415 = call "2_7_Fxp_addation.vi"() -> ()  [unwired: 2 in, 1 out]
  n416 = call "1_7_Fxp_addation.vi"() -> ()  [unwired: 2 in, 1 out]
  n417 = call "16_6_Fxp_addation.vi"() -> ()  [unwired: 2 in, 1 out]
  n418 = call "15_6_Fxp_addation.vi"() -> ()  [unwired: 2 in, 1 out]
  n419 = call "14_6_Fxp_addation.vi"() -> ()  [unwired: 2 in, 1 out]
  n420 = call "13_6_Fxp_addation.vi"() -> ()  [unwired: 2 in, 1 out]
  n421 = call "12_6_Fxp_addation.vi"() -> ()  [unwired: 2 in, 1 out]
  n422 = call "11_6_Fxp_addation.vi"() -> ()  [unwired: 2 in, 1 out]
  n423 = call "10_6_Fxp_addation.vi"() -> ()  [unwired: 2 in, 1 out]
  n424 = call "9_6_Fxp_addation.vi"() -> ()  [unwired: 2 in, 1 out]
  n425 = call "8_6_Fxp_addation.vi"() -> ()  [unwired: 2 in, 1 out]
  n426 = call "7_6_Fxp_addation.vi"() -> ()  [unwired: 2 in, 1 out]
  n427 = call "6_6_Fxp_addation.vi"() -> ()  [unwired: 2 in, 1 out]
  n428 = call "5_6_Fxp_addation.vi"() -> ()  [unwired: 2 in, 1 out]
  n429 = call "4_6_Fxp_addation.vi"() -> ()  [unwired: 2 in, 1 out]
  n430 = call "3_6_Fxp_addation.vi"() -> ()  [unwired: 2 in, 1 out]
  n431 = call "2_6_Fxp_addation.vi"() -> ()  [unwired: 2 in, 1 out]
  n432 = call "1_6_Fxp_addation.vi"() -> ()  [unwired: 2 in, 1 out]
  n433 = call "16_5_Fxp_addation.vi"() -> ()  [unwired: 2 in, 1 out]
  n434 = call "15_5_Fxp_addation.vi"() -> ()  [unwired: 2 in, 1 out]
  n435 = call "14_5_Fxp_addation.vi"() -> ()  [unwired: 2 in, 1 out]
  n436 = call "13_5_Fxp_addation.vi"() -> ()  [unwired: 2 in, 1 out]
  n437 = call "12_5_Fxp_addation.vi"() -> ()  [unwired: 2 in, 1 out]
  n438 = call "11_5_Fxp_addation.vi"() -> ()  [unwired: 2 in, 1 out]
  n439 = call "10_5_Fxp_addation.vi"() -> ()  [unwired: 2 in, 1 out]
  n440 = call "9_5_Fxp_addation.vi"() -> ()  [unwired: 2 in, 1 out]
  n441 = call "8_5_Fxp_addation.vi"() -> ()  [unwired: 2 in, 1 out]
  n442 = call "7_5_Fxp_addation.vi"() -> ()  [unwired: 2 in, 1 out]
  n443 = call "6_5_Fxp_addation.vi"() -> ()  [unwired: 2 in, 1 out]
  n444 = call "5_5_Fxp_addation.vi"() -> ()  [unwired: 2 in, 1 out]
  n445 = call "4_5_Fxp_addation.vi"() -> ()  [unwired: 2 in, 1 out]
  n446 = call "3_5_Fxp_addation.vi"() -> ()  [unwired: 2 in, 1 out]
  n447 = call "2_5_Fxp_addation.vi"() -> ()  [unwired: 2 in, 1 out]
  n448 = call "1_5_Fxp_addation.vi"() -> ()  [unwired: 2 in, 1 out]
  n449 = call "16_4_Fxp_addation.vi"() -> ()  [unwired: 2 in, 1 out]
  n450 = call "15_4_Fxp_addation.vi"() -> ()  [unwired: 2 in, 1 out]
  n451 = call "14_4_Fxp_addation.vi"() -> ()  [unwired: 2 in, 1 out]
  n452 = call "13_4_Fxp_addation.vi"() -> ()  [unwired: 2 in, 1 out]
  n453 = call "12_4_Fxp_addation.vi"() -> ()  [unwired: 2 in, 1 out]
  n454 = call "11_4_Fxp_addation.vi"() -> ()  [unwired: 2 in, 1 out]
  n455 = call "10_4_Fxp_addation.vi"() -> ()  [unwired: 2 in, 1 out]
  n456 = call "9_4_Fxp_addation.vi"() -> ()  [unwired: 2 in, 1 out]
  n457 = call "8_4_Fxp_addation.vi"() -> ()  [unwired: 2 in, 1 out]
  n458 = call "7_4_Fxp_addation.vi"() -> ()  [unwired: 2 in, 1 out]
  n459 = call "6_4_Fxp_addation.vi"() -> ()  [unwired: 2 in, 1 out]
  n460 = call "5_4_Fxp_addation.vi"() -> ()  [unwired: 2 in, 1 out]
  n461 = call "4_4_Fxp_addation.vi"() -> ()  [unwired: 2 in, 1 out]
  n462 = call "3_4_Fxp_addation.vi"() -> ()  [unwired: 2 in, 1 out]
  n463 = call "2_4_Fxp_addation.vi"() -> ()  [unwired: 2 in, 1 out]
  n464 = call "1_4_Fxp_addation.vi"() -> ()  [unwired: 2 in, 1 out]
  n465 = call "16_3_Fxp_addation.vi"() -> ()  [unwired: 2 in, 1 out]
  n466 = call "15_3_Fxp_addation.vi"() -> ()  [unwired: 2 in, 1 out]
  n467 = call "14_3_Fxp_addation.vi"() -> ()  [unwired: 2 in, 1 out]
  n468 = call "13_3_Fxp_addation.vi"() -> ()  [unwired: 2 in, 1 out]
  n469 = call "12_3_Fxp_addation.vi"() -> ()  [unwired: 2 in, 1 out]
  n470 = call "11_3_Fxp_addation.vi"() -> ()  [unwired: 2 in, 1 out]
  n471 = call "10_3_Fxp_addation.vi"() -> ()  [unwired: 2 in, 1 out]
  n472 = call "9_3_Fxp_addation.vi"() -> ()  [unwired: 2 in, 1 out]
  n473 = call "8_3_Fxp_addation.vi"() -> ()  [unwired: 2 in, 1 out]
  n474 = call "7_3_Fxp_addation.vi"() -> ()  [unwired: 2 in, 1 out]
  n475 = call "6_3_Fxp_addation.vi"() -> ()  [unwired: 2 in, 1 out]
  n476 = call "5_3_Fxp_addation.vi"() -> ()  [unwired: 2 in, 1 out]
  n477 = call "4_3_Fxp_addation.vi"() -> ()  [unwired: 2 in, 1 out]
  n478 = call "3_3_Fxp_addation.vi"() -> ()  [unwired: 2 in, 1 out]
  n479 = call "2_3_Fxp_addation.vi"() -> ()  [unwired: 2 in, 1 out]
  n480 = call "1_3_Fxp_addation.vi"() -> ()  [unwired: 2 in, 1 out]
  n481 = call "16_2_Fxp_addation.vi"() -> ()  [unwired: 2 in, 1 out]
  n482 = call "15_2_Fxp_addation.vi"() -> ()  [unwired: 2 in, 1 out]
  n483 = call "14_2_Fxp_addation.vi"() -> ()  [unwired: 2 in, 1 out]
  n484 = call "13_2_Fxp_addation.vi"() -> ()  [unwired: 2 in, 1 out]
  n485 = call "12_2_Fxp_addation.vi"() -> ()  [unwired: 2 in, 1 out]
  n486 = call "11_2_Fxp_addation.vi"() -> ()  [unwired: 2 in, 1 out]
  n487 = call "10_2_Fxp_addation.vi"() -> ()  [unwired: 2 in, 1 out]
  n488 = call "9_2_Fxp_addation.vi"() -> ()  [unwired: 2 in, 1 out]
  n489 = call "8_2_Fxp_addation.vi"() -> ()  [unwired: 2 in, 1 out]
  n490 = call "7_2_Fxp_addation.vi"() -> ()  [unwired: 2 in, 1 out]
  n491 = call "6_2_Fxp_addation.vi"() -> ()  [unwired: 2 in, 1 out]
  n492 = call "5_2_Fxp_addation.vi"() -> ()  [unwired: 2 in, 1 out]
  n493 = call "4_2_Fxp_addation.vi"() -> ()  [unwired: 2 in, 1 out]
  n494 = call "3_2_Fxp_addation.vi"() -> ()  [unwired: 2 in, 1 out]
  n495 = call "2_2_Fxp_addation.vi"() -> ()  [unwired: 2 in, 1 out]
  n496 = call "1_2_Fxp_addation.vi"() -> ()  [unwired: 2 in, 1 out]
  n497 = call "16_1_Fxp_addation.vi"() -> ()  [unwired: 2 in, 1 out]
  n498 = call "15_1_Fxp_addation.vi"() -> ()  [unwired: 2 in, 1 out]
  n499 = call "14_1_Fxp_addation.vi"() -> ()  [unwired: 2 in, 1 out]
  n500 = call "13_1_Fxp_addation.vi"() -> ()  [unwired: 2 in, 1 out]
  n501 = call "12_1_Fxp_addation.vi"() -> ()  [unwired: 2 in, 1 out]
  n502 = call "11_1_Fxp_addation.vi"() -> ()  [unwired: 2 in, 1 out]
  n503 = call "10_1_Fxp_addation.vi"() -> ()  [unwired: 2 in, 1 out]
  n504 = call "9_1_Fxp_addation.vi"() -> ()  [unwired: 2 in, 1 out]
  n505 = call "8_1_Fxp_addation.vi"() -> ()  [unwired: 2 in, 1 out]
  n506 = call "7_1_Fxp_addation.vi"() -> ()  [unwired: 2 in, 1 out]
  n507 = call "6_1_Fxp_addation.vi"() -> ()  [unwired: 2 in, 1 out]
  n508 = call "5_1_Fxp_addation.vi"() -> ()  [unwired: 2 in, 1 out]
  n509 = call "4_1_Fxp_addation.vi"() -> ()  [unwired: 2 in, 1 out]
  n510 = call "3_1_Fxp_addation.vi"() -> ()  [unwired: 2 in, 1 out]
  n511 = call "2_1_Fxp_addation.vi"() -> ()  [unwired: 2 in, 1 out]
  n512 = call "1_1_Fxp_addation.vi"() -> ()  [unwired: 2 in, 1 out]
  n513 = call "FLT_addation.vi"() -> ()  [unwired: 2 in, 1 out]
